vi "MGCC_FntStaMach_FSM loop.vi"() -> (0 "Function":bool[](array[boolean]), 1 "State":bool[](array[boolean]), 4 "Next State":string, 5 "Current State":string)   [LabVIEW 2016]
doc: "This VI is the main loop for the FSM in MGCC. The inputs are the events while the output is the name of the next state."
uses:
  <vilib>/imath/engines/lvmath2/RunTimeEngine/IndexRead/NIMS V(S).vi
  <vilib>/imathl/engines/lvmath/Functions/Error Handling/Create Error.vi
  <vilib>/imath/engines/lvmath2/RunTimeEngine/NodeEndStatement/NIMS_NodeEndStatement_Output.vi
  <vilib>/imath/engines/lvmath2/RunTimeEngine/ErrorHandling/NIMS_Finalize Error.vi
  <vilib>/ErrorRing/Error Ring.xnode
  <vilib>/Utility/error.llb/Error Cluster From Error Code.vi
  Abnormal Fault State Control/Sub_VIs/Fault_Abnormal_state.vi
  Finite State Machine (He Yin)/Sub-VIs/MGCC_FntStaMach_gobal.vi
panel:
  out "error out":errorcluster
  out "error IO":errorcluster
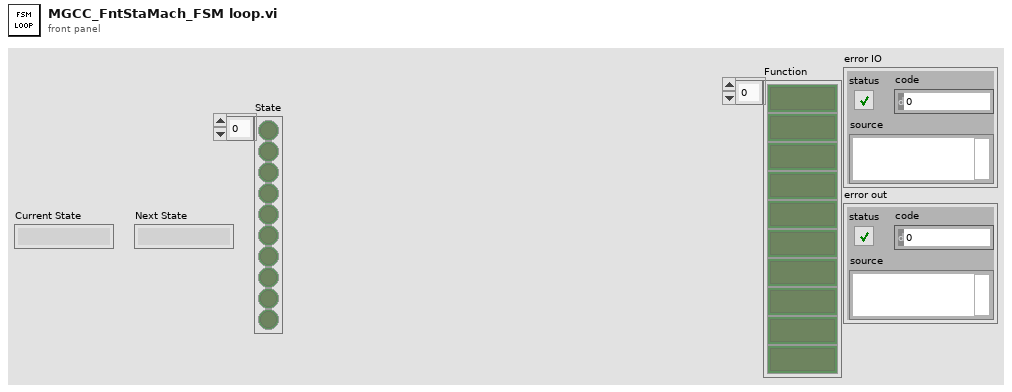
[diagram p1: front panel]
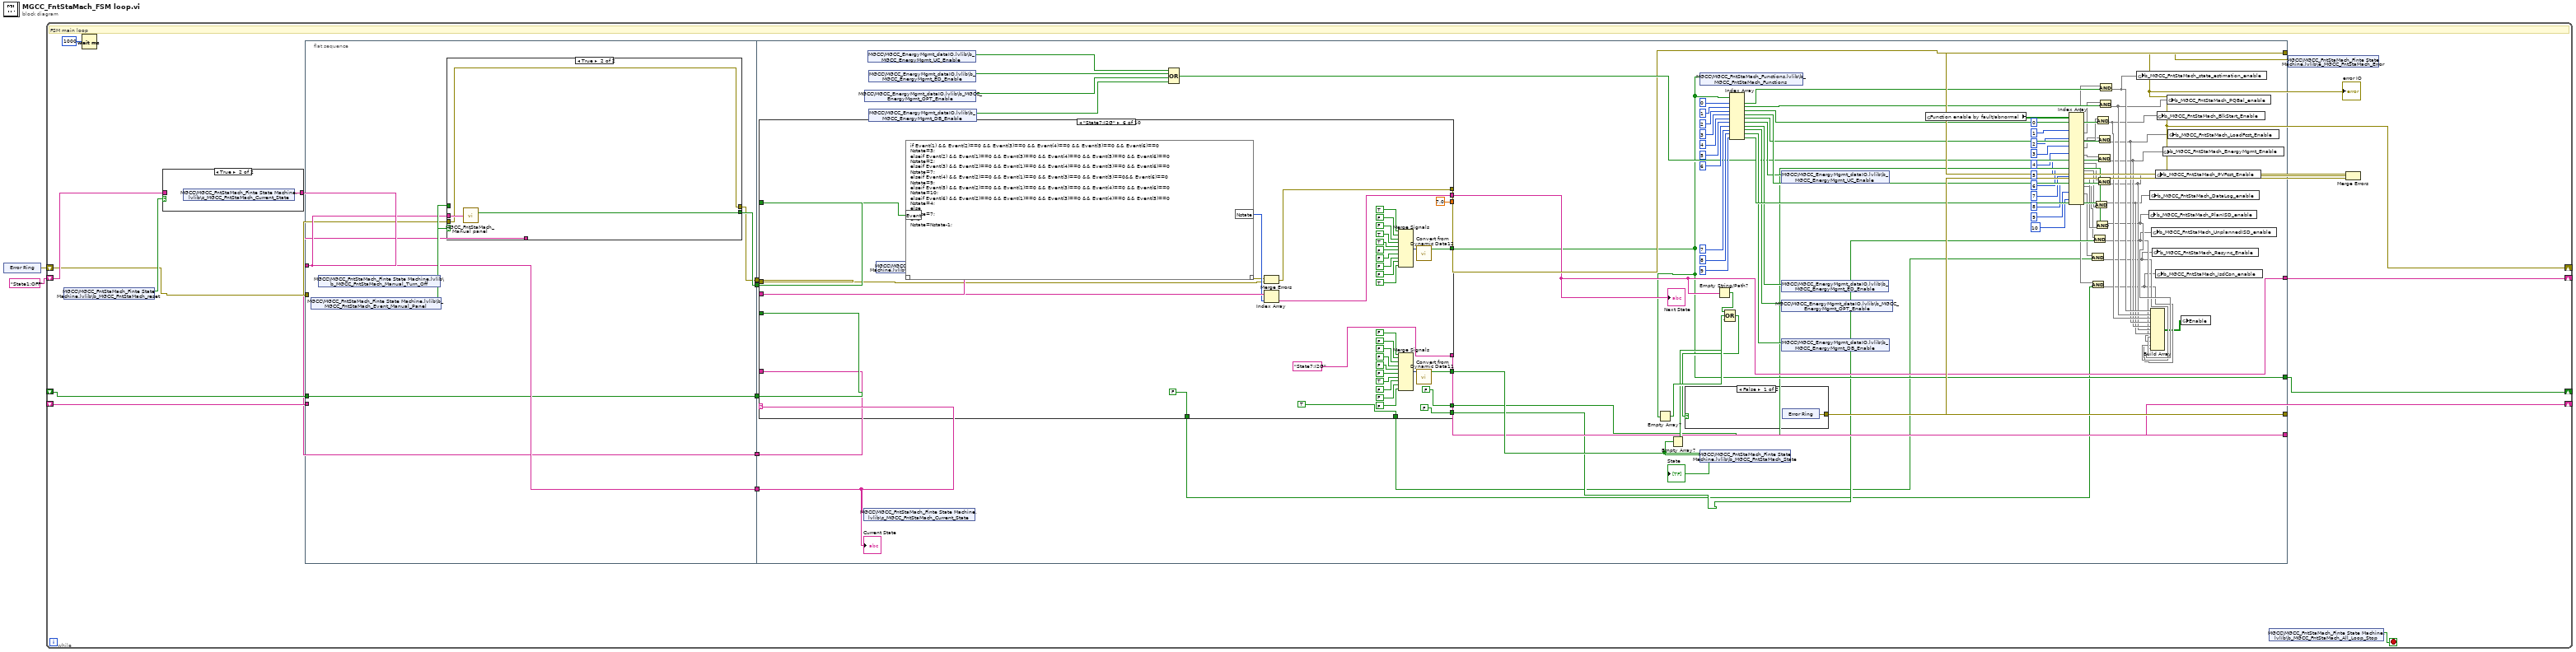
[diagram p0: block diagram]
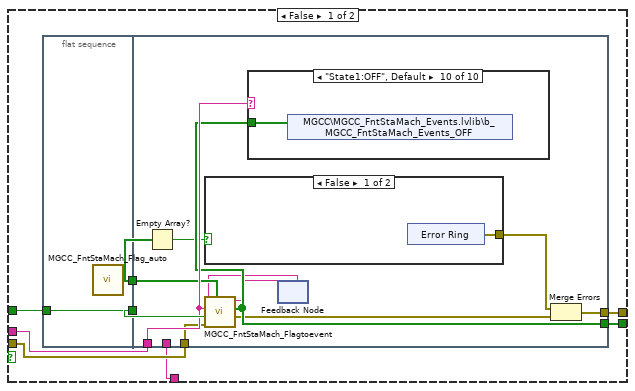
[diagram p3: hidden frame]
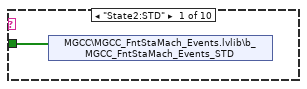
[diagram p4: hidden frame]
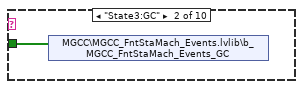
[diagram p5: hidden frame]
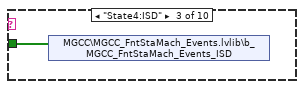
[diagram p6: hidden frame]
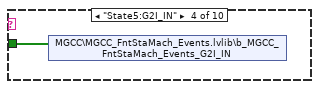
[diagram p7: hidden frame]
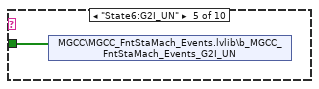
[diagram p8: hidden frame]
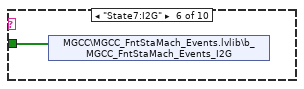
[diagram p9: hidden frame]
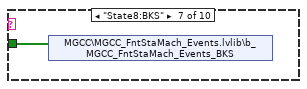
[diagram p10: hidden frame]
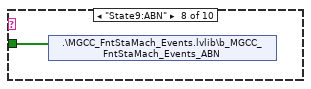
[diagram p11: hidden frame]
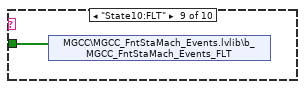
[diagram p12: hidden frame]
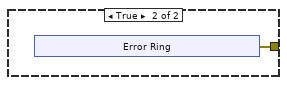
[diagram p13: hidden frame]
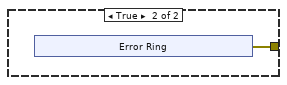
[diagram p14: hidden frame]
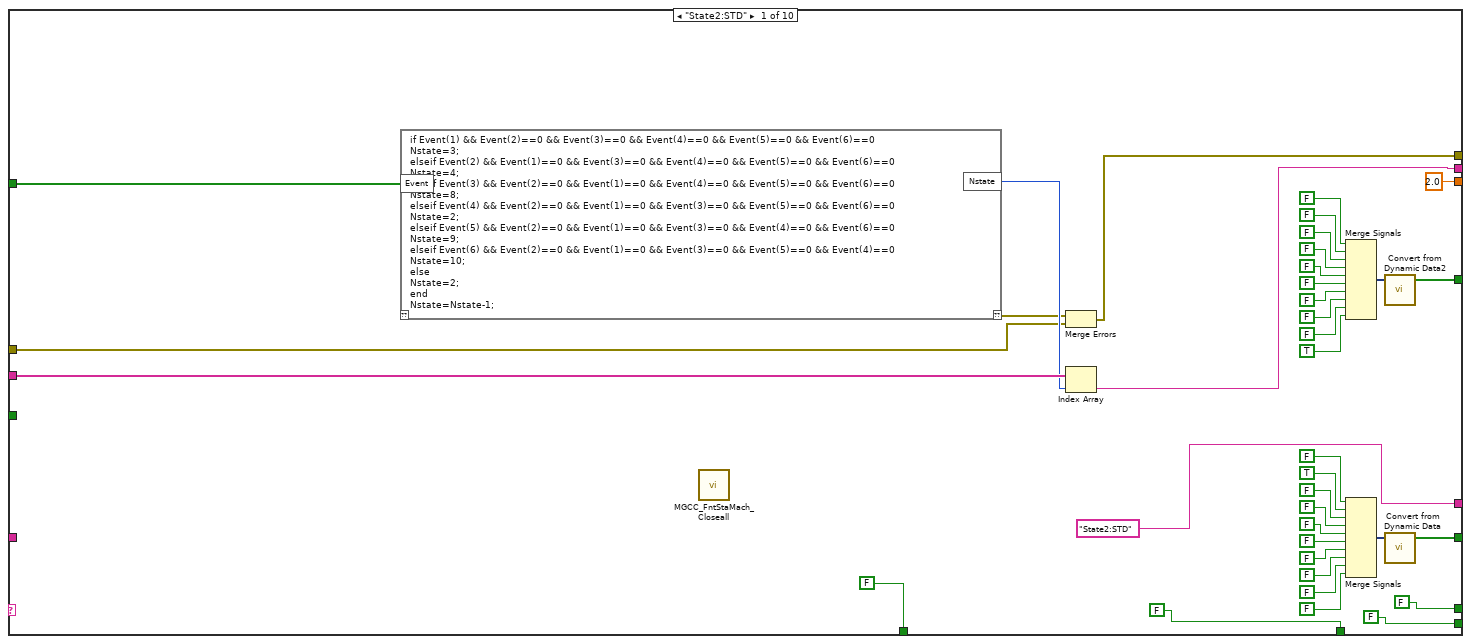
[diagram p15: hidden frame]
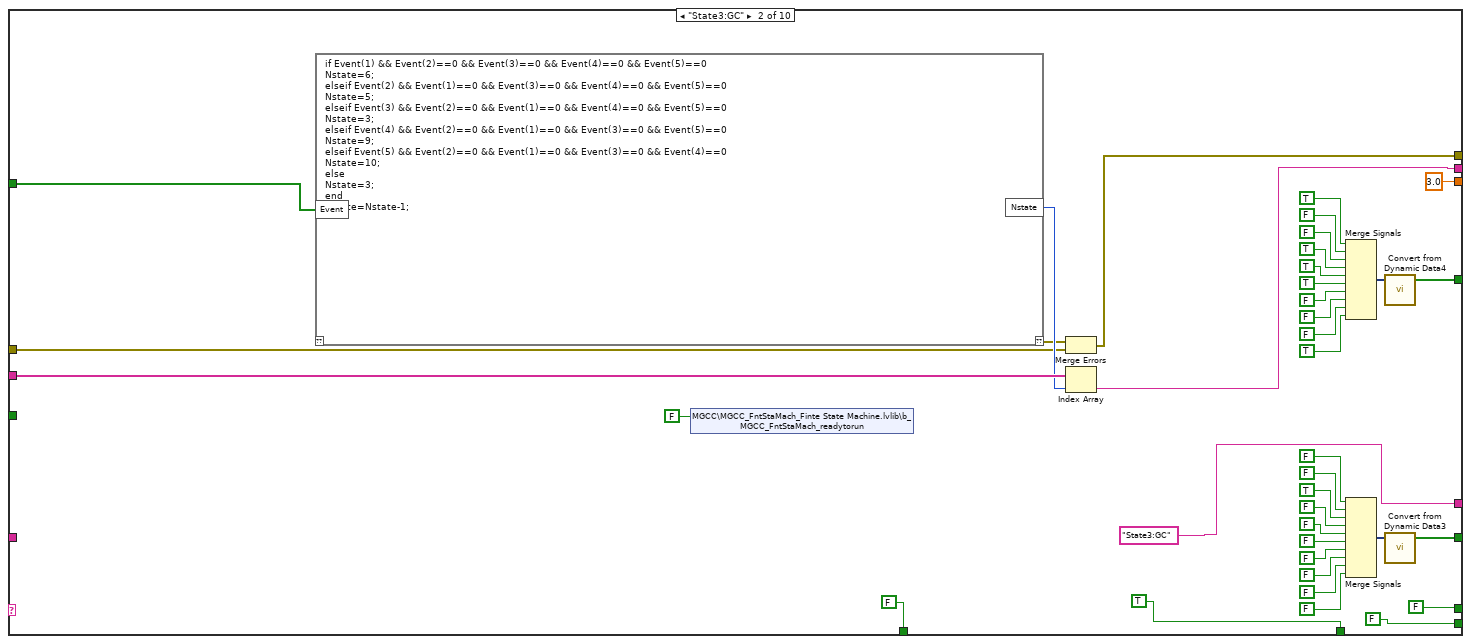
[diagram p16: hidden frame]
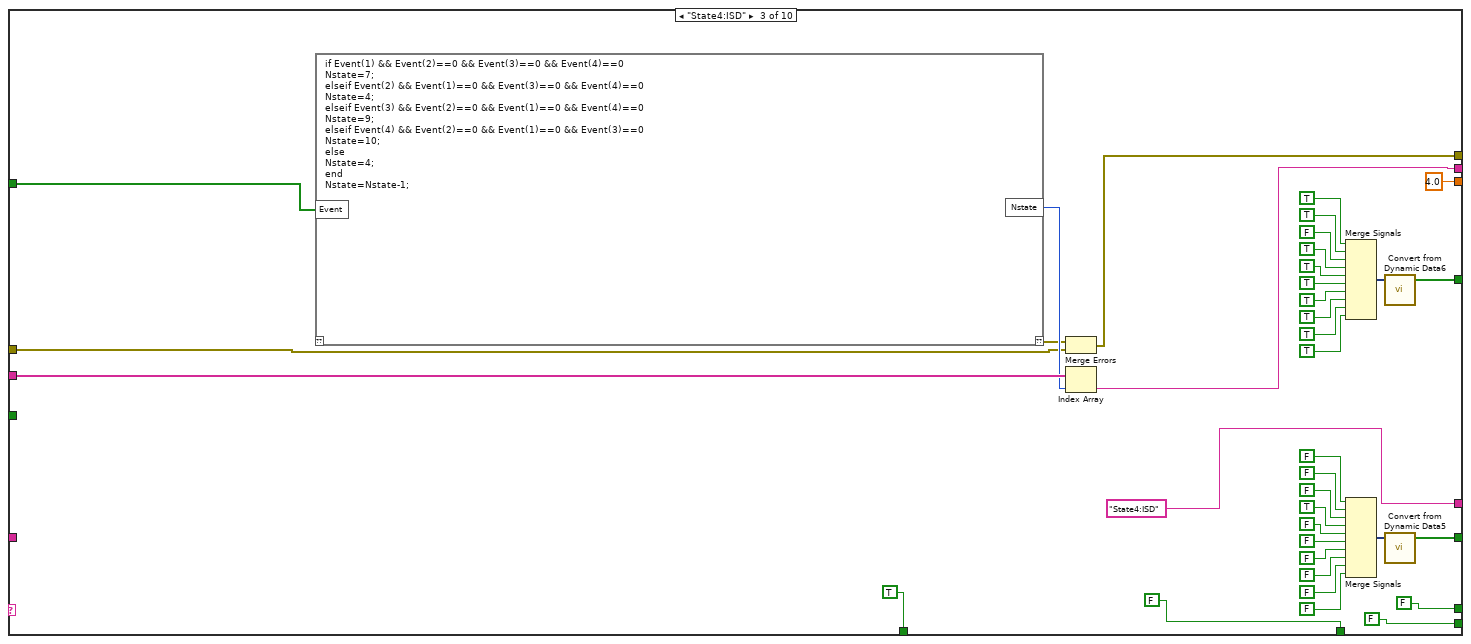
[diagram p17: hidden frame]
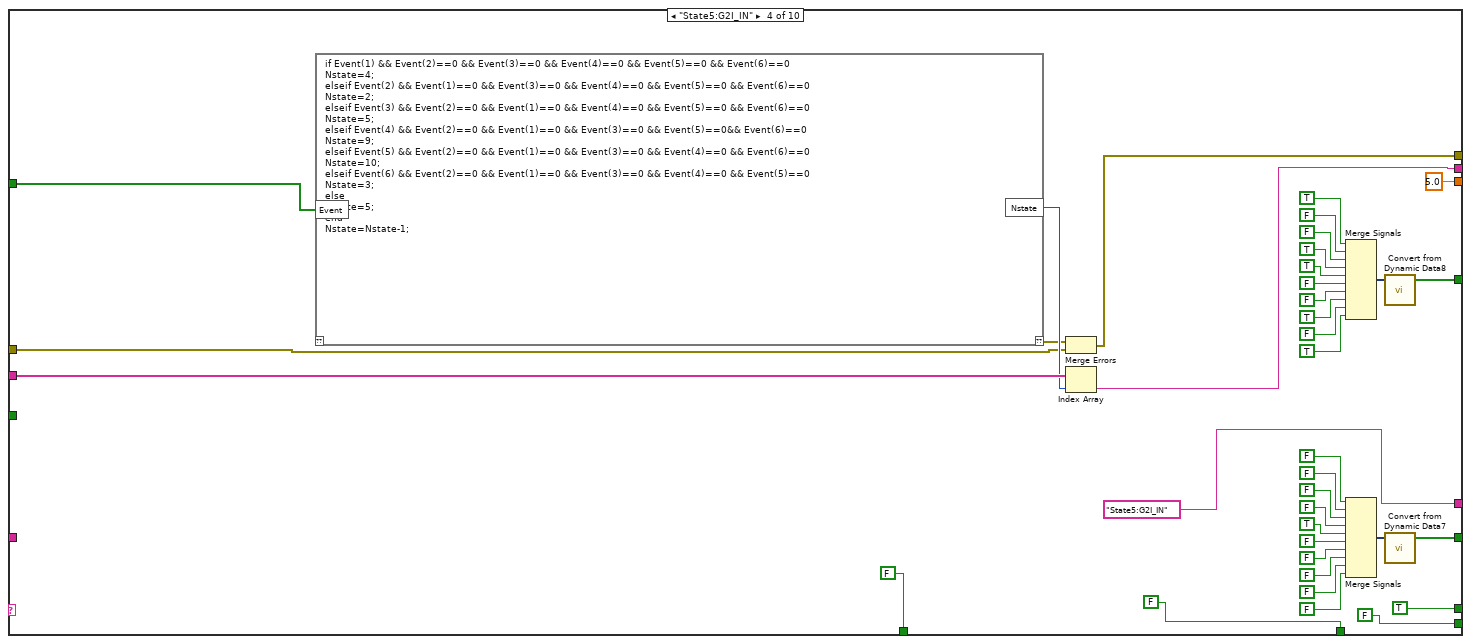
[diagram p18: hidden frame]
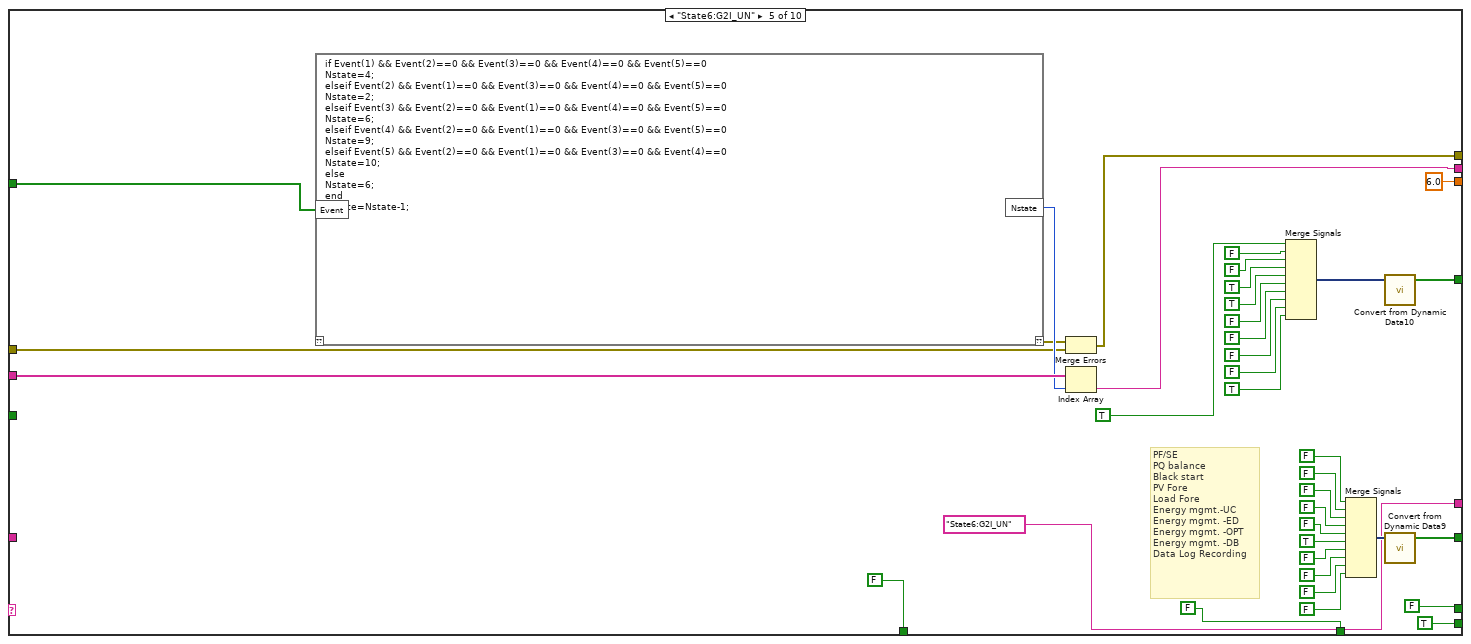
[diagram p19: hidden frame]
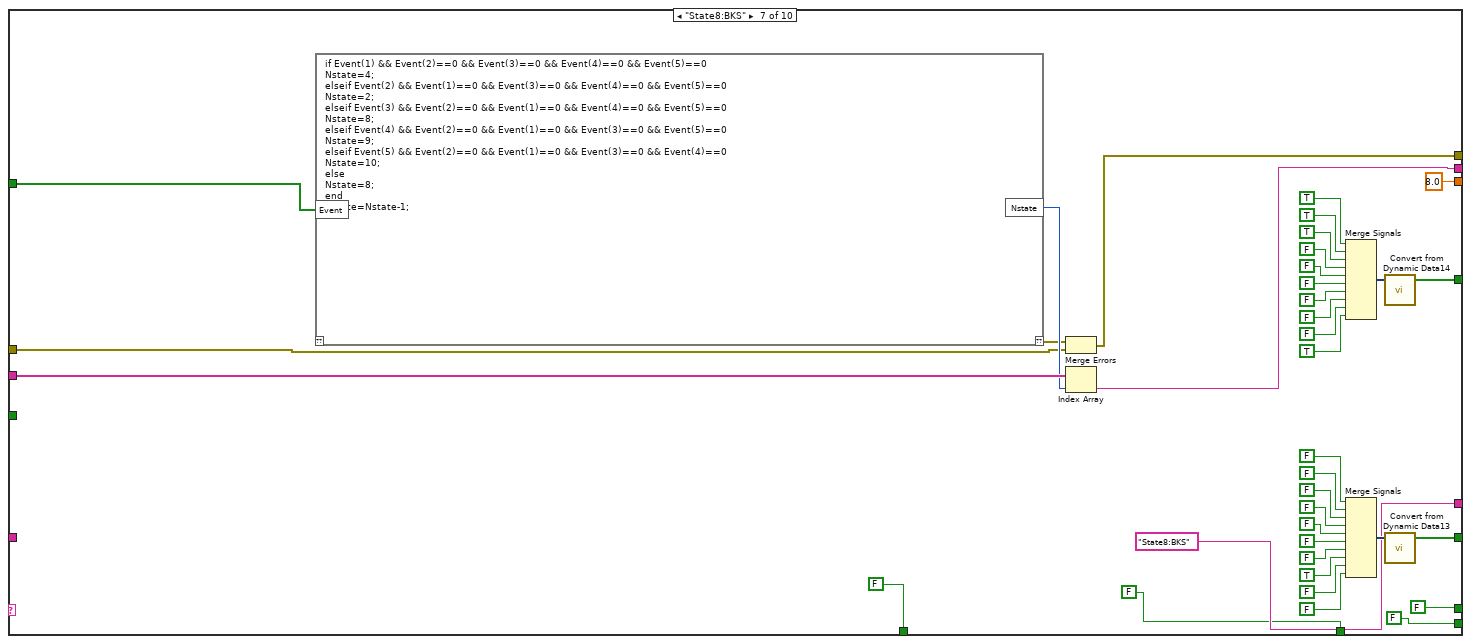
[diagram p20: hidden frame]
diagram:
  n1 = xnode "Error Ring"() -> ("error out"=w1:errorcluster)
  n2 = while {
    shift-right: [w21] -> _
    shift-left: "State1:OFF" ("String") -> [w14]
    shift-right: [w11] -> _
    shift-left: w1 -> [w4]
    shift-right: [w9] -> _
    shift-left: _ -> [w8]
    shift-right: [w7] -> _
    shift-left: _ -> [w5]
    stop <- w19 stop-if-true
    # "FSM main loop"
    n3 = shared-variable "MGCC\\MGCC_FntStaMach_Finte State Machine.lvlib\\b_MGCC_FntStaMach_reset"() -> (w16:bool)  [unwired: 1 in, 1 out]
    n4 = Wait (ms)(milliseconds to wait=u32 1000) -> ()  [unwired: 1 out]
    n5 = case shown="True" w16 {
      tunnel: [w22 w23] -> w15
      tunnel: w14 -> [w22 _]
      frame False {
      }
      frame True {
        n6 = shared-variable "MGCC\\MGCC_FntStaMach_Finte State Machine.lvlib\\s_MGCC_FntStaMach_Current_State"() -> (w23:string)  [unwired: 1 in, 1 out]
      }
    }
    n7 = flat-sequence {
      tunnel: w15 -> [w29]
      tunnel: [w29] -> w18
      tunnel: [w28] -> w17
      tunnel: w4 -> [w27]
      tunnel: [w26] -> w13
      tunnel: w8 -> [w24]
      tunnel: [w25] -> w6
      tunnel: w5 -> [w25]
      tunnel: [w24] -> w3
      tunnel: [w122] -> w21
      tunnel: w18 -> [w152]
      tunnel: w17 -> [w138]
      tunnel: w13 -> [w125]
      tunnel: [w124] -> w12
      tunnel: [w123] -> w10
      tunnel: [w116] -> w9
      tunnel: [w115] -> w7
      tunnel: w6 -> [w114]
      tunnel: w3 -> [w113]
      frame #0 {
        n8 = shared-variable "MGCC\\MGCC_FntStaMach_Finte State Machine.lvlib\\b_MGCC_FntStaMach_Event_Manual_Panel"() -> (w31:bool)  [unwired: 1 in, 1 out]
        n9 = shared-variable "MGCC\\MGCC_FntStaMach_Finte State Machine.lvlib\\b_MGCC_FntStaMach_Manual_Turn_Off"() -> (w30:bool)  [unwired: 1 in, 1 out]
        n10 = case shown="True" w31 {
          tunnel: w30 -> [w39 _]
          tunnel: w29 -> [w37 w73]
          tunnel: [w36 w71] -> w28
          tunnel: w27 -> [w34 w72]
          tunnel: [w33 w72] -> w26
          tunnel: w24 -> [w32 _]
          frame False {
            n11 = flat-sequence {
              tunnel: w39 -> [w41]
              tunnel: [w41] -> w38
              tunnel: [w40] -> w35
              tunnel: w38 -> [w52]
              tunnel: w37 -> [w51]
              tunnel: [w50] -> w36
              tunnel: w35 -> [w48]
              tunnel: w34 -> [w49]
              tunnel: [w44] -> w33
              tunnel: w32 -> [_]
              frame #0 {
                n12 = call "MGCC_FntStaMach_Flag_auto.vi"() -> ("Array"=w40:bool[])
              }
              frame #1 {
                n13 = Empty Array?(array=w48) -> (empty?=w47:bool)
                n14 = case shown="False" w47 {
                  tunnel: [w63 w65] -> w46
                  frame False {
                    n15 = xnode "Error Ring"() -> ("error out"=w63:errorcluster)
                  }
                  frame True {
                    n16 = xnode "Error Ring"() -> ("error out"=w65:errorcluster)
                  }
                }
                n17 = feedback #1() -> (w42:string)  [unwired: 1 in]
                n18 = call "MGCC_FntStaMach_Flagtoevent.vi"("Flags"=w48, "error in"=w49, "M_OFF"=w52, "Pre_state"=w51, "ABN_state"=w42) -> ("error out"=w45:errorcluster, "Event"=w50:bool[], "Previous_state"=w43:string)  [unwired: 4 in]
                n19 = case shown="\"State1:OFF\", Default" w51 {
                  tunnel: w50 -> [w53 w54 w55 w56 w57 w58 w59 w60 w61 w62]
                  frame "State2:STD" {
                    n20 = shared-variable "MGCC\\MGCC_FntStaMach_Events.lvlib\\b_MGCC_FntStaMach_Events_STD"(w53) -> ()  [unwired: 1 in, 1 out]
                  }
                  frame "State3:GC" {
                    n21 = shared-variable "MGCC\\MGCC_FntStaMach_Events.lvlib\\b_MGCC_FntStaMach_Events_GC"(w54) -> ()  [unwired: 1 in, 1 out]
                  }
                  frame "State4:ISD" {
                    n22 = shared-variable "MGCC\\MGCC_FntStaMach_Events.lvlib\\b_MGCC_FntStaMach_Events_ISD"(w55) -> ()  [unwired: 1 in, 1 out]
                  }
                  frame "State5:G2I_IN" {
                    n23 = shared-variable "MGCC\\MGCC_FntStaMach_Events.lvlib\\b_MGCC_FntStaMach_Events_G2I_IN"(w56) -> ()  [unwired: 1 in, 1 out]
                  }
                  frame "State6:G2I_UN" {
                    n24 = shared-variable "MGCC\\MGCC_FntStaMach_Events.lvlib\\b_MGCC_FntStaMach_Events_G2I_UN"(w57) -> ()  [unwired: 1 in, 1 out]
                  }
                  frame "State7:I2G" {
                    n25 = shared-variable "MGCC\\MGCC_FntStaMach_Events.lvlib\\b_MGCC_FntStaMach_Events_I2G"(w58) -> ()  [unwired: 1 in, 1 out]
                  }
                  frame "State8:BKS" {
                    n26 = shared-variable "MGCC\\MGCC_FntStaMach_Events.lvlib\\b_MGCC_FntStaMach_Events_BKS"(w59) -> ()  [unwired: 1 in, 1 out]
                  }
                  frame "State9:ABN" {
                    n27 = shared-variable ".\\MGCC_FntStaMach_Events.lvlib\\b_MGCC_FntStaMach_Events_ABN"(w60) -> ()  [unwired: 1 in, 1 out]
                  }
                  frame "State10:FLT" {
                    n28 = shared-variable "MGCC\\MGCC_FntStaMach_Events.lvlib\\b_MGCC_FntStaMach_Events_FLT"(w61) -> ()  [unwired: 1 in, 1 out]
                  }
                  frame "State1:OFF", Default {
                    n29 = shared-variable "MGCC\\MGCC_FntStaMach_Events.lvlib\\b_MGCC_FntStaMach_Events_OFF"(w62) -> ()  [unwired: 1 in, 1 out]
                  }
                }
                n30 = feedback-in #1(w43) -> ()
                n31 = Merge Errors(w46, w45) -> (w44:errorcluster)
              }
            }
          }
          frame True {
            n32 = call "MGCC_FntStaMach_Manual panel.vi"("current state"=w73) -> ("event"=w71:bool[])
          }
        }
      }
      frame #1 {
        n33 = shared-variable "MGCC\\MGCC_FntStaMach_Finte State Machine.lvlib\\s_MGCC_FntStaMach_Current_State"(w152) -> ()  [unwired: 1 in, 1 out]
        n34 = shared-variable "MGCC\\MGCC_EnergyMgmt_dataIO.lvlib\\b_MGCC_EnergyMgmt_OPT_Enable"() -> (w128:bool)  [unwired: 1 in, 1 out]
        n35 = shared-variable "MGCC\\MGCC_EnergyMgmt_dataIO.lvlib\\b_MGCC_EnergyMgmt_UC_Enable"() -> (w130:bool)  [unwired: 1 in, 1 out]
        n36 = shared-variable "MGCC\\MGCC_EnergyMgmt_dataIO.lvlib\\b_MGCC_EnergyMgmt_ED_Enable"() -> (w129:bool)  [unwired: 1 in, 1 out]
        n37 = shared-variable "MGCC\\MGCC_EnergyMgmt_dataIO.lvlib\\b_MGCC_EnergyMgmt_DB_Enable"() -> (w127:bool)  [unwired: 1 in, 1 out]
        n38 = shared-variable "MGCC\\MGCC_FntStaMach_Finte State Machine.lvlib\\s_MGCC_FntStaMach_State"() -> (w153:string[])  [unwired: 1 in, 1 out]
        n39 = case shown="\"State7:I2G\"" w152 {
          tunnel: [w166 w1154 w1863 w2341 w3329 w4037 w5025 w5735 w7862 w8339] -> w122
          tunnel: [w187 w1176 w1884 w2362 w3350 w4058 w5046 w5754 w7882 w8360] -> w121
          tunnel: w153 -> [w186 w1175 w1883 w2361 w3349 w4057 w5045 w5753 w7881 w8359]
          tunnel: [w174 w1163 w1871 w2349 w3337 w4045 w5034 w5734 w7869 w8347] -> w115
          tunnel: [2.0 ("MS_Analog_Control_OS2_6") 3.0 ("MS_Analog_Control_OS2_6") 4.0 ("MS_Analog_Control_OS2_6") 5.0 ("MS_Analog_Control_OS2_6") 6.0 ("MS_Analog_Control_OS2_6") 7.0 ("MS_Analog_Control_OS2_6") 8.0 ("MS_Analog_Control_OS2_6") 9.0 ("MS_Analog_Control_OS2_6") 10.0 ("MS_Analog_Control_OS2_6") 1.0 ("MS_Analog_Control_OS2_6")] -> _
          tunnel: w138 -> [w171 w1159 w1868 w2346 w3334 w4042 w5030 w5739 w7866 w8344]
          tunnel: w125 -> [w170 w1158 w1867 w2345 w3333 w4041 w5029 w5738 w7865 w8343]
          tunnel: [w168 w1156 w1865 w2343 w3331 w4039 w5027 w5736 w7863 w8341] -> w124
          tunnel: ["State2:STD" "State3:GC" "State4:ISD" "State5:G2I_IN" "State6:G2I_UN" "State7:I2G" "State8:BKS" w5733 "State10:FLT" "State1:OFF"] -> w116
          tunnel: w114 -> [_ _ _ _ _ _ _ w5734 _ _]
          tunnel: w113 -> [_ _ _ _ _ _ _ w5733 _ _]
          tunnel: [FALSE ("State3") FALSE ("State3") FALSE ("State3") TRUE ("State3") FALSE ("State3") FALSE ("State3") FALSE ("State3") FALSE ("State3") FALSE ("State3") FALSE ("State3")] -> w112
          tunnel: [FALSE ("State3") FALSE ("State3") FALSE ("State3") FALSE ("State3") TRUE ("State3") FALSE ("State3") FALSE ("State3") FALSE ("State3") FALSE ("State3") FALSE ("State3")] -> w111
          tunnel: [FALSE ("State3") TRUE ("State3") FALSE ("State3") FALSE ("State3") FALSE ("State3") TRUE ("State3") FALSE ("State3") FALSE ("State3") FALSE ("State3") FALSE ("State3")] -> w74
          tunnel: [FALSE ("State3") FALSE ("State3") TRUE ("State3") FALSE ("State3") FALSE ("State3") FALSE ("State3") FALSE ("State3") FALSE ("State3") FALSE ("State3") FALSE ("State3")] -> w110
          frame "State2:STD" {
            n40 = mathscript code="if Event(1) && Event(2)==0 && Event(3)==0 && Event(4)==0 && Event(5)==0 && Event(6)==0\nNstate=3;\nelseif Event(2) && Event(1)==0 && Event(3)==0 && Event(4)==0 && Event(5)==0 && Event(6)==0\nNstate=4;\nelseif Event(3) && Event(2)==0 && Event(1)==0 && Event(4)==0 && Event(5)==0 && Event(6)==0\nNstate=8;\nelseif Event(4) && Event(2)==0 && Event(1)==0 && Event(3)==0 && Event(5)==0 && Event(6)==0\nNstate=2;\nelseif Event(5) && Event(2)==0 && Event(1)==0 && Event(3)==0 && Event(4)==0 && Event(6)==0\nNstate=9;\nelseif Event(6) && Event(2)==0 && Event(1)==0 && Event(3)==0 && Event(5)==0 && Event(4)==0\nNstate=10;\nelse\nNstate=2;\nend\nNstate=Nstate-1;"("Event"=w171) -> ("??"=w169:errorcluster, "Nstate"=w185:i32)  [unwired: 1 in]
            n41 = call "MGCC_FntStaMach_Closeall.vi"() -> ()  [unwired: 12 in]
            n42 = Merge Errors(w169, w170) -> (w168:errorcluster)
            n43 = Index Array(array=w186, index=w185) -> (element=w166:string)
            n44 = Merge Signals(FALSE ("State3"), FALSE ("State3"), FALSE ("State3"), FALSE ("State3"), FALSE ("State3"), FALSE ("State3"), FALSE ("State3"), FALSE ("State3"), FALSE ("State3"), TRUE ("State3")) -> (w175:dynamicdata)
            n45 = Merge Signals(FALSE ("State3"), TRUE ("State3"), FALSE ("State3"), FALSE ("State3"), FALSE ("State3"), FALSE ("State3"), FALSE ("State3"), FALSE ("State3"), FALSE ("State3"), FALSE ("State3")) -> (w188:dynamicdata)
            n46 = call "Convert from Dynamic Data2"("Dynamic Data Type"=w175) -> ("Array"=w174:bool[])  [unwired: 3 in]
            n47 = call "Convert from Dynamic Data"("Dynamic Data Type"=w188) -> ("Array"=w187:bool[])  [unwired: 3 in]
          }
          frame "State3:GC" {
            n48 = mathscript code="if Event(1) && Event(2)==0 && Event(3)==0 && Event(4)==0 && Event(5)==0 \nNstate=6;\nelseif Event(2) && Event(1)==0 && Event(3)==0 && Event(4)==0 && Event(5)==0 \nNstate=5;\nelseif Event(3) && Event(2)==0 && Event(1)==0 && Event(4)==0 && Event(5)==0 \nNstate=3;\nelseif Event(4) && Event(2)==0 && Event(1)==0 && Event(3)==0 && Event(5)==0\nNstate=9;\nelseif Event(5) && Event(2)==0 && Event(1)==0 && Event(3)==0 && Event(4)==0 \nNstate=10;\nelse\nNstate=3;\nend\nNstate=Nstate-1;"("Event"=w1159) -> ("??"=w1157:errorcluster, "Nstate"=w1174:i32)  [unwired: 1 in]
            n49 = shared-variable "MGCC\\MGCC_FntStaMach_Finte State Machine.lvlib\\b_MGCC_FntStaMach_readytorun"(FALSE ("b_MGCC_DataLog_enable")) -> ()  [unwired: 1 in, 1 out]
            n50 = Merge Errors(w1157, w1158) -> (w1156:errorcluster)
            n51 = Index Array(array=w1175, index=w1174) -> (element=w1154:string)
            n52 = Merge Signals(TRUE ("State3"), FALSE ("State3"), FALSE ("State3"), TRUE ("State3"), TRUE ("State3"), TRUE ("State3"), FALSE ("State3"), FALSE ("State3"), FALSE ("State3"), TRUE ("State3")) -> (w1164:dynamicdata)
            n53 = Merge Signals(FALSE ("State3"), FALSE ("State3"), TRUE ("State3"), FALSE ("State3"), FALSE ("State3"), FALSE ("State3"), FALSE ("State3"), FALSE ("State3"), FALSE ("State3"), FALSE ("State3")) -> (w1177:dynamicdata)
            n54 = call "Convert from Dynamic Data4"("Dynamic Data Type"=w1164) -> ("Array"=w1163:bool[])  [unwired: 3 in]
            n55 = call "Convert from Dynamic Data3"("Dynamic Data Type"=w1177) -> ("Array"=w1176:bool[])  [unwired: 3 in]
          }
          frame "State4:ISD" {
            n56 = mathscript code="if Event(1) && Event(2)==0 && Event(3)==0 && Event(4)==0 \nNstate=7;\nelseif Event(2) && Event(1)==0 && Event(3)==0 && Event(4)==0 \nNstate=4;\nelseif Event(3) && Event(2)==0 && Event(1)==0 && Event(4)==0 \nNstate=9;\nelseif Event(4) && Event(2)==0 && Event(1)==0 && Event(3)==0 \nNstate=10;\nelse\nNstate=4;\nend\nNstate=Nstate-1;"("Event"=w1868) -> ("??"=w1866:errorcluster, "Nstate"=w1882:i32)  [unwired: 1 in]
            n57 = Merge Errors(w1866, w1867) -> (w1865:errorcluster)
            n58 = Index Array(array=w1883, index=w1882) -> (element=w1863:string)
            n59 = Merge Signals(TRUE ("State3"), TRUE ("State3"), FALSE ("State3"), TRUE ("State3"), TRUE ("State3"), TRUE ("State3"), TRUE ("State3"), TRUE ("State3"), TRUE ("State3"), TRUE ("State3")) -> (w1872:dynamicdata)
            n60 = Merge Signals(FALSE ("State3"), FALSE ("State3"), FALSE ("State3"), TRUE ("State3"), FALSE ("State3"), FALSE ("State3"), FALSE ("State3"), FALSE ("State3"), FALSE ("State3"), FALSE ("State3")) -> (w1885:dynamicdata)
            n61 = call "Convert from Dynamic Data6"("Dynamic Data Type"=w1872) -> ("Array"=w1871:bool[])  [unwired: 3 in]
            n62 = call "Convert from Dynamic Data5"("Dynamic Data Type"=w1885) -> ("Array"=w1884:bool[])  [unwired: 3 in]
          }
          frame "State5:G2I_IN" {
            n63 = mathscript code="if Event(1) && Event(2)==0 && Event(3)==0 && Event(4)==0 && Event(5)==0 && Event(6)==0\nNstate=4;\nelseif Event(2) && Event(1)==0 && Event(3)==0 && Event(4)==0 && Event(5)==0 && Event(6)==0\nNstate=2;\nelseif Event(3) && Event(2)==0 && Event(1)==0 && Event(4)==0 && Event(5)==0 && Event(6)==0\nNstate=5;\nelseif Event(4) && Event(2)==0 && Event(1)==0 && Event(3)==0 && Event(5)==0&& Event(6)==0\nNstate=9;\nelseif Event(5) && Event(2)==0 && Event(1)==0 && Event(3)==0 && Event(4)==0 && Event(6)==0\nNstate=10;\nelseif Event(6) && Event(2)==0 && Event(1)==0 && Event(3)==0 && Event(4)==0 && Event(5)==0\nNstate=3;\nelse\nNstate=5;\nend\nNstate=Nstate-1;"("Event"=w2346) -> ("??"=w2344:errorcluster, "Nstate"=w2360:i32)  [unwired: 1 in]
            n64 = Merge Errors(w2344, w2345) -> (w2343:errorcluster)
            n65 = Index Array(array=w2361, index=w2360) -> (element=w2341:string)
            n66 = Merge Signals(TRUE ("State3"), FALSE ("State3"), FALSE ("State3"), TRUE ("State3"), TRUE ("State3"), FALSE ("State3"), FALSE ("State3"), TRUE ("State3"), FALSE ("State3"), TRUE ("State3")) -> (w2350:dynamicdata)
            n67 = Merge Signals(FALSE ("State3"), FALSE ("State3"), FALSE ("State3"), FALSE ("State3"), TRUE ("State3"), FALSE ("State3"), FALSE ("State3"), FALSE ("State3"), FALSE ("State3"), FALSE ("State3")) -> (w2363:dynamicdata)
            n68 = call "Convert from Dynamic Data8"("Dynamic Data Type"=w2350) -> ("Array"=w2349:bool[])  [unwired: 3 in]
            n69 = call "Convert from Dynamic Data7"("Dynamic Data Type"=w2363) -> ("Array"=w2362:bool[])  [unwired: 3 in]
          }
          frame "State6:G2I_UN" {
            # "PF/SE\nPQ balance\nBlack start\nPV Fore\nLoad Fore\nEnergy mgmt.-UC\nEnergy mgmt. -ED\nEnergy mgmt. -OPT\nEnergy mgmt. -DB\nData Log Recording"
            n70 = mathscript code="if Event(1) && Event(2)==0 && Event(3)==0 && Event(4)==0 && Event(5)==0 \nNstate=4;\nelseif Event(2) && Event(1)==0 && Event(3)==0 && Event(4)==0 && Event(5)==0 \nNstate=2;\nelseif Event(3) && Event(2)==0 && Event(1)==0 && Event(4)==0 && Event(5)==0 \nNstate=6;\nelseif Event(4) && Event(2)==0 && Event(1)==0 && Event(3)==0 && Event(5)==0\nNstate=9;\nelseif Event(5) && Event(2)==0 && Event(1)==0 && Event(3)==0 && Event(4)==0 \nNstate=10;\nelse\nNstate=6;\nend\nNstate=Nstate-1;"("Event"=w3334) -> ("??"=w3332:errorcluster, "Nstate"=w3348:i32)  [unwired: 1 in]
            n71 = Merge Errors(w3332, w3333) -> (w3331:errorcluster)
            n72 = Index Array(array=w3349, index=w3348) -> (element=w3329:string)
            n73 = Merge Signals(TRUE ("State3"), FALSE ("State3"), FALSE ("State3"), TRUE ("State3"), TRUE ("State3"), FALSE ("State3"), FALSE ("State3"), FALSE ("State3"), FALSE ("State3"), TRUE ("State3")) -> (w3338:dynamicdata)
            n74 = Merge Signals(FALSE ("State3"), FALSE ("State3"), FALSE ("State3"), FALSE ("State3"), FALSE ("State3"), TRUE ("State3"), FALSE ("State3"), FALSE ("State3"), FALSE ("State3"), FALSE ("State3")) -> (w3351:dynamicdata)
            n75 = call "Convert from Dynamic Data10"("Dynamic Data Type"=w3338) -> ("Array"=w3337:bool[])  [unwired: 3 in]
            n76 = call "Convert from Dynamic Data9"("Dynamic Data Type"=w3351) -> ("Array"=w3350:bool[])  [unwired: 3 in]
          }
          frame "State7:I2G" {
            n77 = mathscript code="if Event(1) && Event(2)==0 && Event(3)==0 && Event(4)==0 && Event(5)==0 && Event(6)==0 \nNstate=3;\nelseif Event(2) && Event(1)==0 && Event(3)==0 && Event(4)==0 && Event(5)==0 && Event(6)==0 \nNstate=2;\nelseif Event(3) && Event(2)==0 && Event(1)==0 && Event(4)==0 && Event(5)==0 && Event(6)==0 \nNstate=7;\nelseif Event(4) && Event(2)==0 && Event(1)==0 && Event(3)==0 && Event(5)==0&& Event(6)==0 \nNstate=9;\nelseif Event(5) && Event(2)==0 && Event(1)==0 && Event(3)==0 && Event(4)==0 && Event(6)==0 \nNstate=10;\nelseif Event(6) && Event(2)==0 && Event(1)==0 && Event(3)==0 && Event(4)==0 && Event(5)==0 \nNstate=4;\nelse\nNstate=7;\nend\nNstate=Nstate-1;"("Event"=w4042) -> ("??"=w4040:errorcluster, "Nstate"=w4056:i32)  [unwired: 1 in]
            n78 = Merge Errors(w4040, w4041) -> (w4039:errorcluster)
            n79 = Index Array(array=w4057, index=w4056) -> (element=w4037:string)
            n80 = Merge Signals(TRUE ("State3"), FALSE ("State3"), FALSE ("State3"), TRUE ("State3"), TRUE ("State3"), FALSE ("State3"), FALSE ("State3"), FALSE ("State3"), FALSE ("State3"), TRUE ("State3")) -> (w4046:dynamicdata)
            n81 = Merge Signals(FALSE ("State3"), FALSE ("State3"), FALSE ("State3"), FALSE ("State3"), FALSE ("State3"), FALSE ("State3"), TRUE ("State3"), FALSE ("State3"), FALSE ("State3"), FALSE ("State3")) -> (w4059:dynamicdata)
            n82 = call "Convert from Dynamic Data12"("Dynamic Data Type"=w4046) -> ("Array"=w4045:bool[])  [unwired: 3 in]
            n83 = call "Convert from Dynamic Data11"("Dynamic Data Type"=w4059) -> ("Array"=w4058:bool[])  [unwired: 3 in]
          }
          frame "State8:BKS" {
            n84 = mathscript code="if Event(1) && Event(2)==0 && Event(3)==0 && Event(4)==0 && Event(5)==0 \nNstate=4;\nelseif Event(2) && Event(1)==0 && Event(3)==0 && Event(4)==0 && Event(5)==0 \nNstate=2;\nelseif Event(3) && Event(2)==0 && Event(1)==0 && Event(4)==0 && Event(5)==0 \nNstate=8;\nelseif Event(4) && Event(2)==0 && Event(1)==0 && Event(3)==0 && Event(5)==0\nNstate=9;\nelseif Event(5) && Event(2)==0 && Event(1)==0 && Event(3)==0 && Event(4)==0 \nNstate=10;\nelse\nNstate=8;\nend\nNstate=Nstate-1;"("Event"=w5030) -> ("??"=w5028:errorcluster, "Nstate"=w5031:i32)  [unwired: 1 in]
            n85 = Merge Errors(w5028, w5029) -> (w5027:errorcluster)
            n86 = Index Array(array=w5045, index=w5031) -> (element=w5025:string)
            n87 = Merge Signals(TRUE ("State3"), TRUE ("State3"), TRUE ("State3"), FALSE ("State3"), FALSE ("State3"), FALSE ("State3"), FALSE ("State3"), FALSE ("State3"), FALSE ("State3"), TRUE ("State3")) -> (w5035:dynamicdata)
            n88 = Merge Signals(FALSE ("State3"), FALSE ("State3"), FALSE ("State3"), FALSE ("State3"), FALSE ("State3"), FALSE ("State3"), FALSE ("State3"), TRUE ("State3"), FALSE ("State3"), FALSE ("State3")) -> (w5047:dynamicdata)
            n89 = call "Convert from Dynamic Data14"("Dynamic Data Type"=w5035) -> ("Array"=w5034:bool[])  [unwired: 3 in]
            n90 = call "Convert from Dynamic Data13"("Dynamic Data Type"=w5047) -> ("Array"=w5046:bool[])  [unwired: 3 in]
          }
          frame "State9:ABN" {
            n91 = mathscript code="if Event(1) && Event(2)==0 && Event(3)==0 && Event(4)==0 && Event(5)==0 && Event(6)==0 && Event(7)==0 && Event(8)==0 && Event(9)==0 \nNstate=2;\nelseif Event(2) && Event(1)==0 && Event(3)==0 && Event(4)==0 && Event(5)==0 && Event(6)==0 && Event(7)==0 && Event(8)==0 && Event(9)==0 \nNstate=3;\nelseif Event(3) && Event(2)==0 && Event(1)==0 && Event(4)==0 && Event(5)==0 && Event(6)==0 && Event(7)==0 && Event(8)==0 && Event(9)==0 \nNstate=4;\nelseif Event(4) && Event(2)==0 && Event(1)==0 && Event(3)==0 && Event(5)==0&& Event(6)==0 && Event(7)==0 && Event(8)==0 && Event(9)==0 \nNstate=6;\nelseif Event(5) && Event(2)==0 && Event(1)==0 && Event(3)==0 && Event(4)==0 && Event(6)==0 && Event(7)==0 && Event(8)==0 && Event(9)==0 \nNstate=5;\nelseif Event(6) && Event(2)==0 && Event(1)==0 && Event(3)==0 && Event(4)==0 && Event(5)==0 && Event(7)==0 && Event(8)==0 && Event(9)==0 \nNstate=7;\nelseif Event(7) && Event(2)==0 && Event(1)==0 && Event(3)==0 && Event(4)==0 && Event(6)==0 && Event(5)==0 && Event(8)==0 && Event(9)==0 \nNstate=8;\nelseif Event(8) && Event(2)==0 && Event(1)==0 && Event(3)==0 && Event(4)==0 && Event(6)==0 && Event(7)==0 && Event(5)==0 && Event(9)==0 \nNstate=9;\nelseif Event(9) && Event(2)==0 && Event(1)==0 && Event(3)==0 && Event(4)==0 && Event(6)==0 && Event(7)==0 && Event(8)==0 && Event(5)==0 \nNstate=10;\nelse\nNstate=9;\nend\nNstate=Nstate-1;"("Event"=w5739) -> ("??"=w5737:errorcluster, "Nstate"=w5752:i32)  [unwired: 1 in]
            "error out" <- w5737
            n92 = Index Array(array=w5753, index=w5752) -> (element=w5735:string)
            n93 = Merge Errors(w5737, w5738) -> (w5736:errorcluster)
            n94 = Merge Signals(TRUE ("State3"), TRUE ("State3"), TRUE ("State3"), TRUE ("State3"), TRUE ("State3"), TRUE ("State3"), TRUE ("State3"), TRUE ("State3"), TRUE ("State3"), TRUE ("State3")) -> (w5742:dynamicdata)
            n95 = Merge Signals(FALSE ("State3"), FALSE ("State3"), FALSE ("State3"), FALSE ("State3"), FALSE ("State3"), FALSE ("State3"), FALSE ("State3"), FALSE ("State3"), TRUE ("State3"), FALSE ("State3")) -> (w5755:dynamicdata)
            n96 = call "Convert from Dynamic Data16"("Dynamic Data Type"=w5742) -> ()  [unwired: 3 in, 1 out]
            n97 = call "Convert from Dynamic Data15"("Dynamic Data Type"=w5755) -> ("Array"=w5754:bool[])  [unwired: 3 in]
          }
          frame "State10:FLT" {
            n98 = mathscript code="if Event(1) && Event(2)==0 && Event(3)==0 && Event(4)==0 \nNstate=10;\nelseif Event(2) && Event(1)==0 && Event(3)==0 && Event(4)==0 \nNstate=9;\nelseif Event(3) && Event(2)==0 && Event(1)==0 && Event(4)==0 \nNstate=2;\nelseif Event(4) && Event(2)==0 && Event(1)==0 && Event(3)==0 \nNstate=1;\nelse\nNstate=10;\nend\nNstate=Nstate-1;"("Event"=w7866) -> ("??"=w7864:errorcluster, "Nstate"=w7880:i32)  [unwired: 1 in]
            n99 = Merge Errors(w7864, w7865) -> (w7863:errorcluster)
            n100 = Index Array(array=w7881, index=w7880) -> (element=w7862:string)
            n101 = Merge Signals(FALSE ("State3"), FALSE ("State3"), FALSE ("State3"), FALSE ("State3"), FALSE ("State3"), FALSE ("State3"), FALSE ("State3"), FALSE ("State3"), FALSE ("State3"), TRUE ("State3")) -> (w7870:dynamicdata)
            n102 = Merge Signals(FALSE ("State3"), FALSE ("State3"), FALSE ("State3"), FALSE ("State3"), FALSE ("State3"), FALSE ("State3"), FALSE ("State3"), FALSE ("State3"), FALSE ("State3"), TRUE ("State3")) -> (w7883:dynamicdata)
            n103 = call "Convert from Dynamic Data18"("Dynamic Data Type"=w7870) -> ("Array"=w7869:bool[])  [unwired: 3 in]
            n104 = call "Convert from Dynamic Data17"("Dynamic Data Type"=w7883) -> ("Array"=w7882:bool[])  [unwired: 3 in]
          }
          frame "State1:OFF", Default {
            # "The relationship between the events and the states can be find\nin the Q2 report."
            # "This FSM is used to determine the working state of MGCC FSM. The input are the events in each state while the outputs are the next states. If error events happens, it will stay in the current state."
            n105 = disable-structure shown="Disabled" {
              frame Disabled {
                n106 = shared-variable "MGCC\\MGCC_FntStaMach_Finte State Machine.lvlib\\b_MGCC_FntStaMach_readytorun"(TRUE ("b_MGCC_DataLog_enable")) -> ()  [unwired: 1 in, 1 out]
              }
              frame Enabled {
              }
            }
            n107 = mathscript code="if Event(1) && Event(2)==0 && Event(3)==0\nNstate=2;\nelseif Event(2) && Event(1)==0 && Event(3)==0\nNstate=9;\nelseif Event(3) && Event(2)==0 && Event(1)==0\nNstate=10;\nelse\nNstate=1;\nend\nNstate=Nstate-1;"("Event"=w8344) -> ("??"=w8342:errorcluster, "Nstate"=w8358:i32)  [unwired: 1 in]
            n108 = Merge Errors(w8342, w8343) -> (w8341:errorcluster)
            n109 = Index Array(array=w8359, index=w8358) -> (element=w8339:string)
            n110 = Merge Signals(FALSE ("State3"), FALSE ("State3"), FALSE ("State3"), FALSE ("State3"), FALSE ("State3"), FALSE ("State3"), FALSE ("State3"), FALSE ("State3"), FALSE ("State3"), FALSE ("State3")) -> (w8348:dynamicdata)
            n111 = Merge Signals(TRUE ("State3"), FALSE ("State3"), FALSE ("State3"), FALSE ("State3"), FALSE ("State3"), FALSE ("State3"), FALSE ("State3"), FALSE ("State3"), FALSE ("State3"), FALSE ("State3")) -> (w8361:dynamicdata)
            n112 = call "Convert from Dynamic Data20"("Dynamic Data Type"=w8348) -> ("Array"=w8347:bool[])  [unwired: 3 in]
            n113 = call "Convert from Dynamic Data19"("Dynamic Data Type"=w8361) -> ("Array"=w8360:bool[])  [unwired: 3 in]
          }
        }
        "Next State" <- w122
        "State" <- w121
        n114 = Compound Arithmetic op=OR(w130, w129, w128, w127) -> (w126:bool)
        n115 = Empty Array?(array=w115) -> (empty?=w120:bool)
        n116 = Empty Array?(array=w121) -> (empty?=w119:bool)
        n117 = shared-variable "MGCC\\MGCC_FntStaMach_Functions.lvlib\\b_MGCC_FntStaMach_Functions"(w115) -> ()  [unwired: 1 in, 1 out]
        n118 = shared-variable "MGCC\\MGCC_FntStaMach_Finte State Machine.lvlib\\b_MGCC_FntStaMach_State"(w121) -> ()  [unwired: 1 in, 1 out]
        n119 = Empty String/Path?(string/path=w122) -> (empty?=w118:bool)
        n120 = Compound Arithmetic op=OR(w118, w120, w119) -> (w117:bool)
        n121 = case shown="False" w117 {
          tunnel: [w154 w156] -> w123
          frame False {
            n122 = xnode "Error Ring"() -> ("error out"=w154:errorcluster)
          }
          frame True {
            n123 = xnode "Error Ring"() -> ("error out"=w156:errorcluster)
          }
        }
        n124 = Index Array(array=w115, index #1=0 ("index"), index #2=1 ("index"), index #3=2 ("index"), index #4=3 ("index"), index #5=4 ("index"), index #6=5 ("index"), index #7=6 ("index"), index #8=7 ("index"), index #9=8 ("index"), index #10=9 ("index")) -> (element #1=w137:bool, element #2=w141:bool, element #3=w140:bool, element #4=w136:bool, element #5=w135:bool, element #6=w134:bool, element #7=w133:bool, element #8=w132:bool, element #9=w131:bool, element #10=w139:bool)
        n125 = shared-variable "MGCC\\MGCC_EnergyMgmt_dataIO.lvlib\\b_MGCC_EnergyMgmt_UC_Enable"(w134) -> ()  [unwired: 1 in, 1 out]
        n126 = shared-variable "MGCC\\MGCC_EnergyMgmt_dataIO.lvlib\\b_MGCC_EnergyMgmt_ED_Enable"(w133) -> ()  [unwired: 1 in, 1 out]
        n127 = shared-variable "MGCC\\MGCC_EnergyMgmt_dataIO.lvlib\\b_MGCC_EnergyMgmt_OPT_Enable"(w132) -> ()  [unwired: 1 in, 1 out]
        n128 = shared-variable "MGCC\\MGCC_EnergyMgmt_dataIO.lvlib\\b_MGCC_EnergyMgmt_DB_Enable"(w131) -> ()  [unwired: 1 in, 1 out]
        n129 = global read "Fault_Abnormal_state.vi" "Function enable by fault/abnormal"() -> (w109:bool[][])
        n130 = Index Array(array=w109, index (row) #1=0 ("index"), index (row) #2=1 ("index"), index (row) #3=2 ("index"), index (row) #4=3 ("index"), index (row) #5=4 ("index"), index (row) #6=5 ("index"), index (row) #7=6 ("index"), index (row) #8=7 ("index"), index (row) #9=8 ("index"), index (row) #10=9 ("index"), index (row) #11=10 ("index")) -> (element #1=w97:bool[], element #2=w96:bool[], element #3=w95:bool[], element #4=w94:bool[], element #5=w93:bool[], element #6=w92:bool[], element #7=w91:bool[], element #8=w90:bool[], element #9=w89:bool[], element #10=w88:bool[], element #11=w87:bool[])  [unwired: 11 in]
        n131 = And(x=w88, y=w74) -> (x .and. y?=w77:bool[])
        n132 = And(x=w87, y=w110) -> (x .and. y?=w76:bool[])
        n133 = And(x=w89, y=w111) -> (x .and. y?=w78:bool[])
        n134 = And(x=w139, y=w91) -> (x .and. y?=w80:bool[])
        n135 = And(x=w112, y=w90) -> (x .and. y?=w79:bool[])
        n136 = And(x=w95, y=w140) -> (x .and. y?=w84:bool[])
        n137 = And(x=w93, y=w126) -> (x .and. y?=w82:bool[])
        n138 = And(x=w92, y=w136) -> (x .and. y?=w81:bool[])
        n139 = And(x=w94, y=w135) -> (x .and. y?=w83:bool[])
        n140 = And(x=w96, y=w141) -> (x .and. y?=w85:bool[])
        n141 = And(x=w97, y=w137) -> (x .and. y?=w86:bool[])
        n142 = global write "MGCC_FntStaMach_gobal.vi" "b_MGCC_FntStaMach_state_estimation_enable"(w86) -> ()
        n143 = global write "MGCC_FntStaMach_gobal.vi" "b_MGCC_FntStaMach_PlanISD_enable"(w79) -> ()
        n144 = global write "MGCC_FntStaMach_gobal.vi" "b_MGCC_FntStaMach_DataLog_enable"(w80) -> ()
        n145 = Build Array(w86, w85, w84, w83, w82, w81, w80, w79, w78, w77, w76) -> (w75:bool[][])
        n146 = global write "MGCC_FntStaMach_gobal.vi" "b_MGCC_FntStaMach_UnplannedISD_enable"(w78) -> ()
        n147 = global write "MGCC_FntStaMach_gobal.vi" "b_MGCC_FntStaMach_Resync_Enable"(w77) -> ()
        n148 = global write "MGCC_FntStaMach_gobal.vi" "b_MGCC_FntStaMach_PVFcst_Enable"(w81) -> ()
        n149 = global write "MGCC_FntStaMach_gobal.vi" "b_MGCC_FntStaMach_IsdCon_enable"(w76) -> ()
        n150 = global write "MGCC_FntStaMach_gobal.vi" "b_MGCC_FntStaMach_BlkStart_Enable"(w84) -> ()
        n151 = global write "MGCC_FntStaMach_gobal.vi" "b_MGCC_FntStaMach_EnergyMgmt_Enable"(w82) -> ()
        n152 = global write "MGCC_FntStaMach_gobal.vi" "b_MGCC_FntStaMach_PQBal_enable"(w85) -> ()
        n153 = global write "MGCC_FntStaMach_gobal.vi" "b_MGCC_FntStaMach_LoadFcst_Enable"(w83) -> ()
        n154 = global write "MGCC_FntStaMach_gobal.vi" "Enable"(w75) -> ()
        "Current State" <- w152
      }
    }
    n155 = shared-variable "MGCC\\MGCC_FntStaMach_Finte State Machine.lvlib\\b_MGCC_FntStaMach_All_Loop_Stop"() -> (w19:bool)  [unwired: 1 in, 1 out]
    n156 = Merge Errors(w12, w10) -> (w11:errorcluster)
    "error IO" <- w11
    n157 = shared-variable "MGCC\\MGCC_FntStaMach_Finte State Machine.lvlib\\e_MGCC_FntStaMach_Error"(w11) -> ()  [unwired: 1 in, 1 out]
  }
